vi "Hide.vi"(6 "L/T":bool, 8 "iterations":i32=319, 9 "Image Pixels In (U8)":u8[][](array[numeric])) -> (0 "static":u8[][](array[numeric]), 4 "hide":bool)   [LabVIEW 2015]
uses:
  TypeDefs Host/Open Audio FGV Enum.ctl
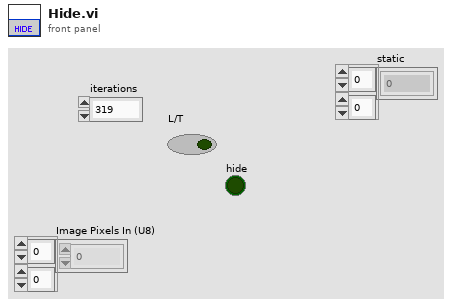
[diagram p1: front panel]
types:
  T1 = typedef "Open Audio FGV Enum.ctl" = enum16{"Get", "Set"}
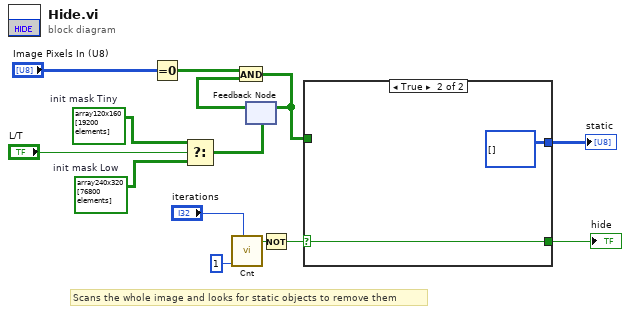
[diagram p0: block diagram]
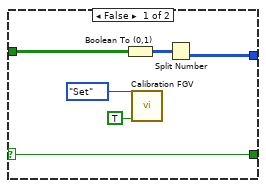
[diagram p2: hidden frame]
diagram:
  w5 = bool[][] array240x320[76800 elements]  # init mask Low
  w6 = bool[][] array120x160[19200 elements]  # init mask Tiny
  # "Scans the whole image and looks for static objects to remove them"
  n1 = Equal To 0?(x="Image Pixels In (U8)") -> (x = 0?=w9:bool[][])
  n2 = Select(t=w6, s="L/T", f=w5) -> (s? t:f=w7:bool[][])
  n3 = call "Cnt.vi"("n-1"="iterations", "inc"=1) -> ("end"=w3:bool)  [unwired: 8 in, 1 out]
  n4 = feedback #1(w7) -> (w8:bool[][])
  n5 = And(x=w9, y=w8) -> (x .and. y?=w1:bool[][])
  n6 = feedback-in #1(w1) -> ()
  n7 = Not(x=w3) -> (.not. x?=w2:bool)
  n8 = case shown="True" w2 {
    selector: w2 -> [w19 w22]
    tunnel: [w19 w22] -> w14
    tunnel: [w17 u8[][] []] -> w13
    tunnel: w1 -> [w18 _]
    frame False {
      n9 = Boolean To (0,1)(Boolean=w18) -> (0, 1=w20:i16[][])
      n10 = call "Calibration FGV.vi"("Command"=Open_Audio_FGV_Enum."Set", "Calib"=TRUE) -> ()  [unwired: 9 in, 1 out]
      n11 = Split Number(x=w20) -> (lo(x)=w17:u8[][])  [unwired: 1 out]
    }
    frame True {
    }
  }
  "hide" <- w14
  "static" <- w13
